vi "DoE_Control_v6.vi"() -> ()   [LabVIEW 2015]
uses:
  --Sensor and Instrument Drivers--/LabView VI Drivers for Heise DXD Digital Pressure Transducer/Type Defs/DXD Address.ctl
  --Controls and TypeDefs--/DoE_Control_Cluster.ctl
panel:
  out "Data Cluster 2":T1={"Current DoE"=[], "SSI 1 Flow Rate"=0.0, "SSI 2 Flow Rate"=0.0, "FLOM 1 Flow Rate"=0.0, "FLOM 2 Flow Rate"=0.0, "Pumps Running?"=FALSE, "Boolean 2"=FALSE, "Boolean 3"=FALSE, "Boolean 4"=FALSE, "At Equilibrium?"=FALSE, "Script Running?"=FALSE, "Current Script Iteration"=0.0, "Total Script Iterations"=0.0, "FLOM Pumps VISA"="COM2", "SSI 1 Pump VISA"="COM76", "SSI 2 Pump VISA"="COM74", "Huber Unistat VISA"="COM1", "SSI 3 Pump VISA"="COM76", "SSI 4 Pump VISA"="COM76", "SSI 4 Flow Rate"=0.0, "SSI 3 Flow Rate"=0.0, "Flow Meter 1"="COM76", "Flow Meter 2"="COM76", "Flow Meter 3"="COM76", "Flow Meter 4"="COM76", "Flow Meter 1 Rate "=0.0, "Flow Meter 2 Rate"=0.0, "Flow Meter 3 Rate"=0.0, "Flow Meter 4 Rate"=0.0, "SSI 1 Flow Setpoint"=0.0, "SSI 2 Flow Setpoint"=0.0, "SSI 3 Flow Setpoint"=0.0, "SSI 4 Flow Setpoint"=0.0, "Temperature Setpoint"=0.0} {"Current DoE" format="%0.3f"}
  in  "Sensor Readouts":T2(tab)
  out "Thermocouple T-Plots":cluster{dbl, dbl, dbl}(graph)
  in  "Flow meter 1 COM":u16=15
  in  "Flow meter 2 COM":u16=16
  in  "Flow meter 4 COM":u16=19
  in  "Flow meter 5 COM":u16=18
  out "Flow Rate":T3(graph)
  in  "Flow meter 3 COM":u16=17
  out "Temp":T4(graph)
  out "Pressure":T5(graph)
  in  "Pressure COM":refnum<visa-resource-name>="COM6"
  in  "Unit":T6(ring)
  in  "Write to File?":bool
  in  "?":T7(tab)
  in  "Collect Spectra":bool
  out "Raman Spectrum":cluster{i32[], i32[]}[](graph)
  in  "Reset?":bool
  in  "Cancel Script":bool
  in  "Data Cluster":T1={"Current DoE"=[], "SSI 1 Flow Rate"=0.0, "SSI 2 Flow Rate"=0.0, "FLOM 1 Flow Rate"=0.0, "FLOM 2 Flow Rate"=0.0, "Pumps Running?"=FALSE, "Boolean 2"=FALSE, "Boolean 3"=FALSE, "Boolean 4"=FALSE, "At Equilibrium?"=FALSE, "Script Running?"=FALSE, "Current Script Iteration"=0.0, "Total Script Iterations"=0.0, "FLOM Pumps VISA"="COM2", "SSI 1 Pump VISA"="COM76", "SSI 2 Pump VISA"="COM74", "Huber Unistat VISA"="COM1", "SSI 3 Pump VISA"="COM76", "SSI 4 Pump VISA"="COM76", "SSI 4 Flow Rate"=0.0, "SSI 3 Flow Rate"=0.0, "Flow Meter 1"="COM76", "Flow Meter 2"="COM76", "Flow Meter 3"="COM76", "Flow Meter 4"="COM76", "Flow Meter 1 Rate "=0.0, "Flow Meter 2 Rate"=0.0, "Flow Meter 3 Rate"=0.0, "Flow Meter 4 Rate"=0.0, "SSI 1 Flow Setpoint"=0.0, "SSI 2 Flow Setpoint"=0.0, "SSI 3 Flow Setpoint"=0.0, "SSI 4 Flow Setpoint"=0.0, "Temperature Setpoint"=0.0} {"Current DoE" format="%0.3f"}
  in  "?":T8(tab)
  in  "Huber Unistat VISA":refnum<visa-resource-name>="COM1"
  in  "SSI 4 Pump VISA":refnum<visa-resource-name>="COM10"
  in  "SSI 2 Pump VISA 2":refnum<visa-resource-name>="COM8"
  in  "SSI 1 Pump VISA":refnum<visa-resource-name>="COM7"
  in  "FLOM Pumps VISA":refnum<visa-resource-name>="LPT1"
  in  "SSI 3 Pump VISA":refnum<visa-resource-name>="COM9"
  in  "Set COMs":bool
  out "Data_noRaman path":path caption="selected path"
  out "Data_Reactant 1 path":path caption="selected path"
  out "Data_Product path":path caption="selected path"
  out "Data_Reactant 3 path":path caption="selected path"
  out "Data_Reactant 2 path":path caption="selected path"
  out "Raman Data Path":T9
  in  "Create DoE":bool
  out "file write cancelled":bool caption="cancelled"
  out "written file already exists (and overwritten)":bool caption="exists"
  in  "Input DoE Values":string[][](table)
  in  "Load DoE":bool
  out "Current DoE":dbl[][](array[numeric]) format="%0.3f"
  out "DoE Filename":path
  in  "Get Current DoE":bool
  in  "Stop-Start SSI 4":bool
  in  "Stop-Start SSI 3":bool
  in  "Edit or Run/Stop SSI 4":string(combo)="Run/Stop"
  in  "Edit or Run/Stop SSI 3":string(combo)="Run/Stop"
  in  "Pump 4 (Green)?":bool
  in  "Pump 3 (Yellow)?":bool
  in  "SSI  4 (Green)":dbl
  in  "SSI  3 (Yellow)":dbl
  in  "SSI  1 (Red)":dbl
  in  "Manual Pump Control?":bool
  in  "SSI  2 (Blue)":dbl
  in  "Pump 1 (Red)?":bool
  in  "Pump 2 (Blue)?":bool
  in  "Edit or Run/Stop SSI 2":string(combo)="Run/Stop"
  in  "Edit or Run/Stop SSI 1":string(combo)="Run/Stop"
  in  "Stop-Start SSI 1":bool
  in  "Stop-Start SSI 2":bool
  in  "FLOM 1":dbl min=0.0 max=9900.0 step=1.0
  in  "FLOM 2":dbl min=0.0 max=9900.0 step=1.0
  in  "FLOM 1?":bool
  in  "FLOM 2?":bool
  in  "Stop   Start FLOM 1":bool
  in  "Stop   Start FLOM 2":bool
  in  "Edit Values, or Run Flow? FLOM 2":string(combo)="Run/Stop"
  in  "Edit Values, or Run Flow? FLOM 1":string(combo)="Run/Stop"
  out "SSI  2  (Blue) Feedback":i32 format="%.2f"
  out "SSI  1  (Red) Feedback":i32 format="%.2f"
  out "SSI  3  (Yellow) Feedback":i32 format="%.2f"
  out "SSI  4  (Green) Feedback":i32 format="%.2f"
  in  "Set Temp / Lower Limit / Upper Limit":dbl
  in  "Manual Temp Control?":bool
  out "Last Command Written":string="Upper limit is"
  out "Temperature Output":string="Upper limit is"
  out "Last Message from Pump":string="Heating pump message, 2:38:53 PM:\nTemperature is set to 0.000000K"
  out "Error Out":T10
  in  "Commands":string(combo)="Setup"
  in  "Run Current DoE":bool
  out "Last Message from Pump":string="Heating pump message, 2:38:53 PM:\nTemperature is set to 0.000000K"
  out "Current Experiment":dbl[](array[numeric])
  in  "Debugging / Send Command":string
  in  "Debug":bool
  out "Program State":string
  in  "?":bool
  # "Most recent update: 2/23/2016 - JMW"
  # "Features To-Implement:\n\n- Yield Plotting and Analytics\n- Feedback Control based on Yield\n- Error Generation System\n     - for system and user safety"
  # "Notes:\n- set upper and lower temperature limits using \"Manual Temp Control\" \n     - DoE can't access T values outside of these limits\n- repeatedly turning the temperature control on and off can lead to compressor wear - avoid!\n- Added T and P readouts and saving\n- Always use Stop Program rather than the LabView stop button, else the Sensirion DLL\n   calls will error out and LabView must be restarted"
  # "Not corrrect com, set later"
  # "SSI 1"
  # "SSI 2"
  # "SSI 3"
  # "SSI 4"
  # "Temp"
  # "Time"
  # "FLOM 1"
  # "FLOM 2"
  # "SSI 1"
  # "SSI 2"
  # "SSI 3"
  # "SSI 4"
  # "FLOM 1"
  # "FLOM 2"
  # "Temp"
  # "Time"
  # "All flow rates in increments of 10uL/min"
  # "Note: don't repeatedly turn off and on temperature control as this can wear out the compressor too rapidly according to Unistat\nManual"
  # "Time"
  # "Temp"
  # "SSI 1"
  # "SSI 2"
  # "SSI 3"
  # "SSI 4"
  # "FLOM 1"
  # "FLOM 2"
  # "uL/min , degrees C, seconds"
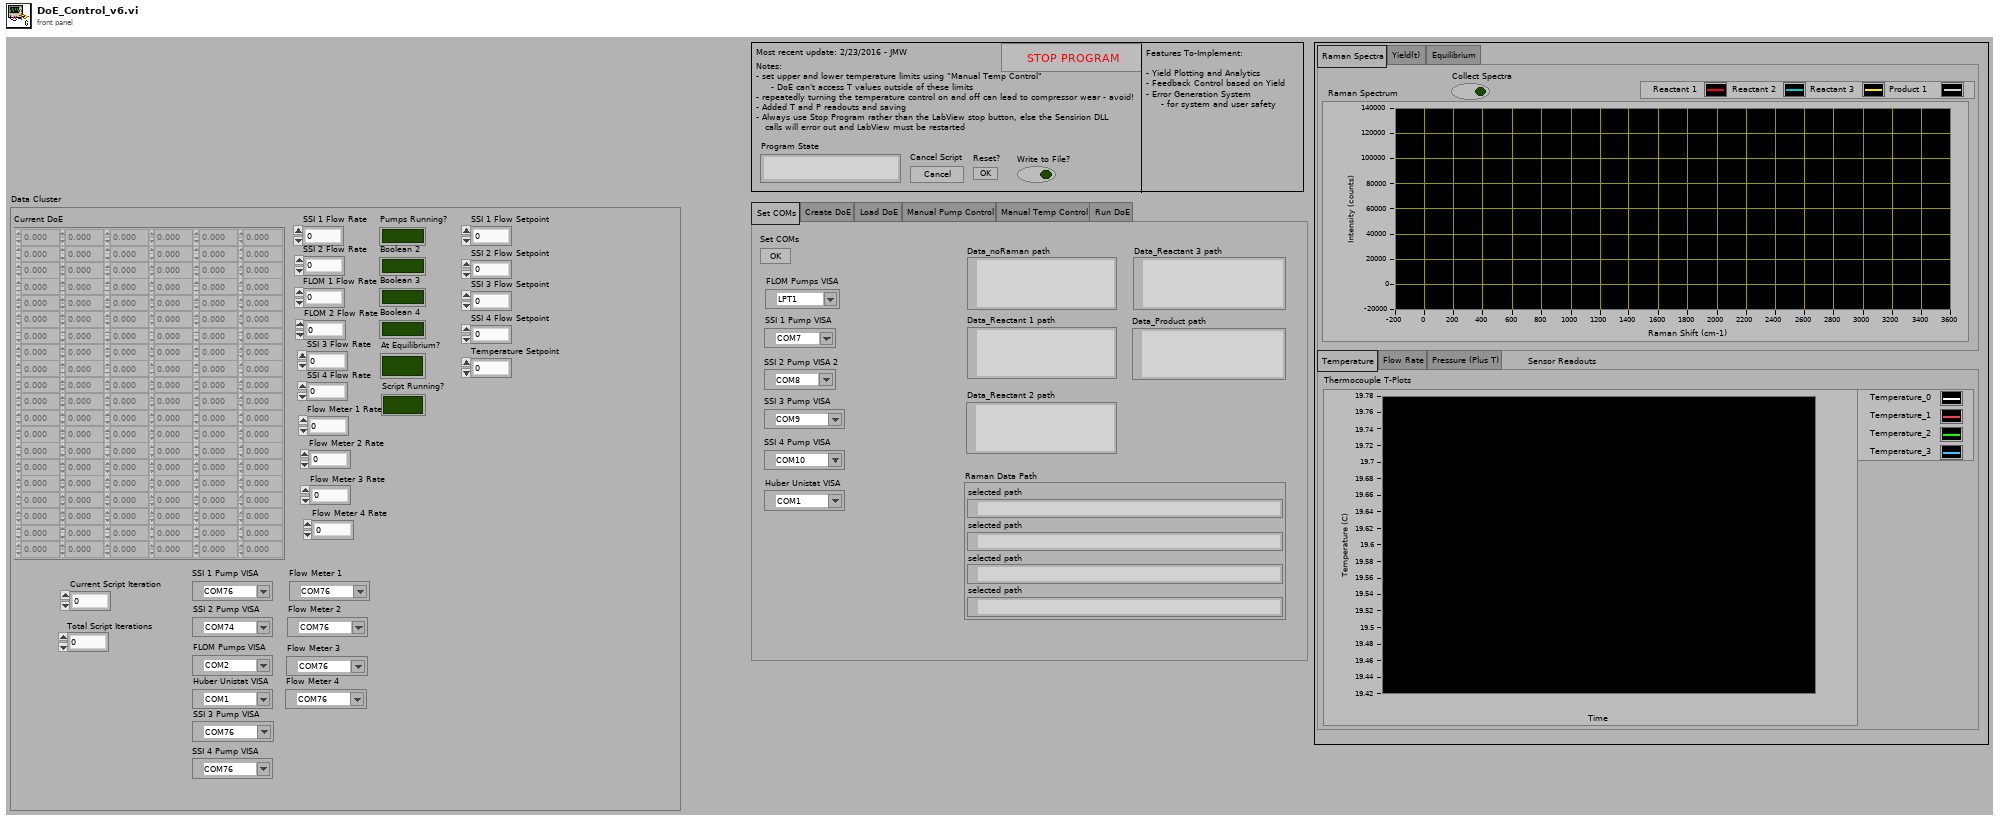
[diagram p1: front panel]
types:
  T1 = typedef "DoE_Control_Cluster.ctl" = cluster{"Current DoE":dbl[][], "SSI 1 Flow Rate":dbl, "SSI 2 Flow Rate":dbl, "FLOM 1 Flow Rate":dbl, "FLOM 2 Flow Rate":dbl, "Pumps Running?":bool, "Boolean 2":bool, "Boolean 3":bool, "Boolean 4":bool, "At Equilibrium?":bool, "Script Running?":bool, "Current Script Iteration":dbl, "Total Script Iterations":dbl, "FLOM Pumps VISA":refnum<visa-resource-name>, "SSI 1 Pump VISA":refnum<visa-resource-name>, "SSI 2 Pump VISA":refnum<visa-resource-name>, "Huber Unistat VISA":refnum<visa-resource-name>, "SSI 3 Pump VISA":refnum<visa-resource-name>, "SSI 4 Pump VISA":refnum<visa-resource-name>, "SSI 4 Flow Rate":dbl, "SSI 3 Flow Rate":dbl, "Flow Meter 1":refnum<visa-resource-name>, "Flow Meter 2":refnum<visa-resource-name>, "Flow Meter 3":refnum<visa-resource-name>, "Flow Meter 4":refnum<visa-resource-name>, "Flow Meter 1 Rate ":dbl, "Flow Meter 2 Rate":dbl, "Flow Meter 3 Rate":dbl, "Flow Meter 4 Rate":dbl, "SSI 1 Flow Setpoint":dbl, "SSI 2 Flow Setpoint":dbl, "SSI 3 Flow Setpoint":dbl, "SSI 4 Flow Setpoint":dbl, "Temperature Setpoint":dbl}
  T2 = enum32{"Temperature", "Flow Rate", "Pressure (Plus T)"}
  T3 = cluster{"MeasureResult Scaled":dbl, "MeasureResult Scaled":dbl, "MeasureResult Scaled":dbl, "MeasureResult Scaled":dbl, "MeasureResult Scaled":dbl}
  T4 = cluster{"Current Temperature":dbl, "Current Temperature":dbl, "Current Temperature":dbl, "Current Temperature":dbl}
  T5 = cluster{"Current Pressure":dbl, "Current Pressure":dbl, "Current Pressure":dbl, "Current Pressure":dbl}
  T6 = enum16{"PSI", "Bar", "cm H2O", "ft H2O", "hectoPascal", "in Hg", "in H2O", "kiloPascal", "milliBar", "mmHg", "MegaPascal", "Numeric Pressure"}
  T7 = enum32{"Raman Spectra", "Yield(t)", "Equilibrium"}
  T8 = enum32{"Set COMs", "Create DoE", "Load DoE", "Manual Pump Control", "Manual Temp Control", "Run DoE"}
  T9 = cluster{"selected path":path, "selected path":path, "selected path":path, "selected path":path}
  T10 = cluster{"status":bool, "code":i32, "Error Report":string}
  T11 = cluster{"Array":dbl[], "Array 2":dbl[], "Array 3":dbl[], "Array 4":dbl[], "Array 5":dbl[]}
  T12 = cluster{"MeasureResult Scaled":dbl, "MeasureResult Scaled":dbl, "MeasureResult Scaled":dbl, "MeasureResult Scaled":dbl, "MeasureResult Scaled":dbl}[]
  T13 = cluster{"appended path":path, "appended path":path, "appended path":path, "appended path":path, "appended path":path}
  T14 = cluster{"Current Pressure":dbl, "Current Pressure":dbl, "Current Pressure":dbl, "Current Pressure":dbl}[]
  T15 = cluster{"Current Temperature":dbl, "Current Temperature":dbl, "Current Temperature":dbl, "Current Temperature":dbl}[]
  T16 = typedef "DXD Address.ctl" = i32
  T17 = cluster{"Data_noRaman path":path, "Data_Reactant 1 path":path, "Data_Reactant 2 path":path, "Data_Reactant 3 path":path, "Data_Product path":path}
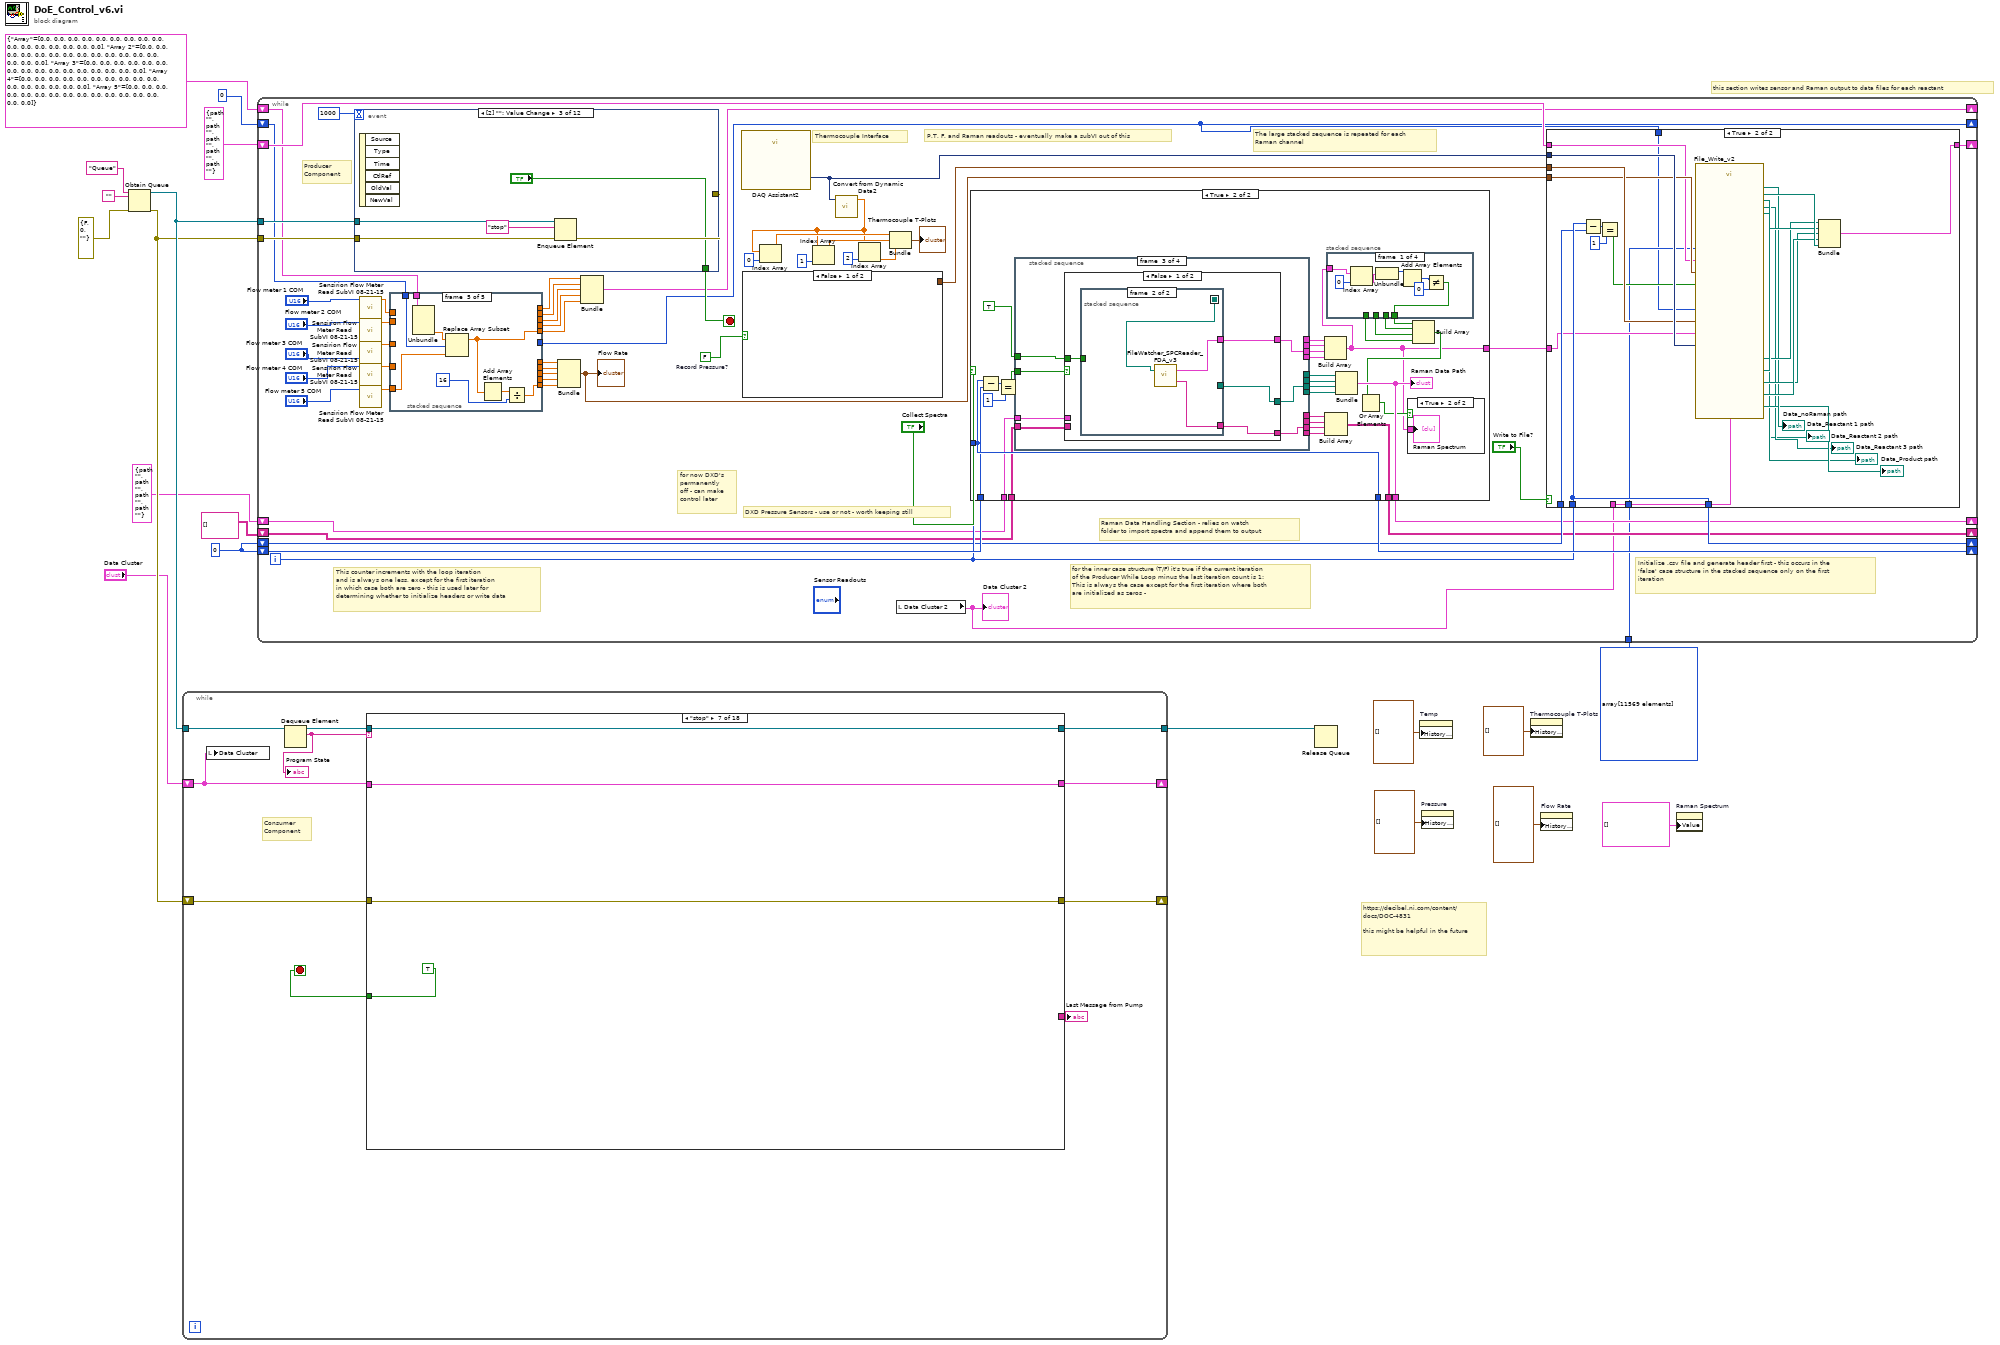
[diagram p0: block diagram]
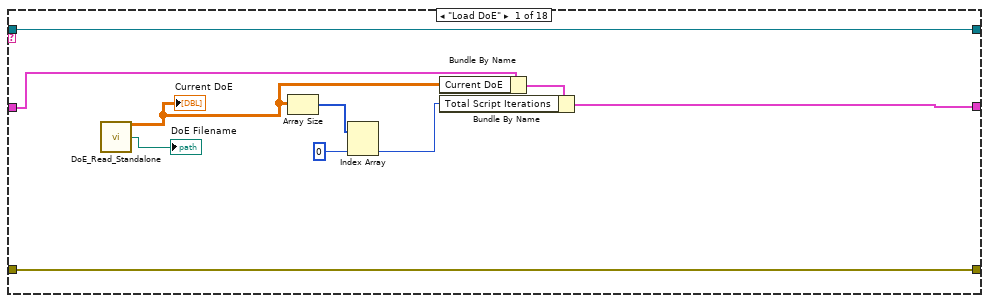
[diagram p2: hidden frame]
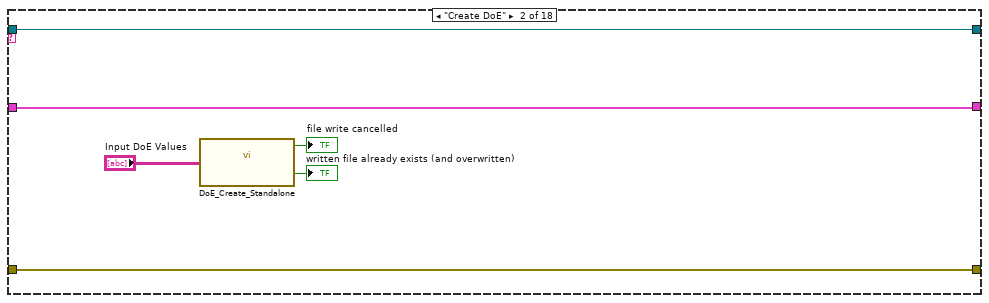
[diagram p3: hidden frame]
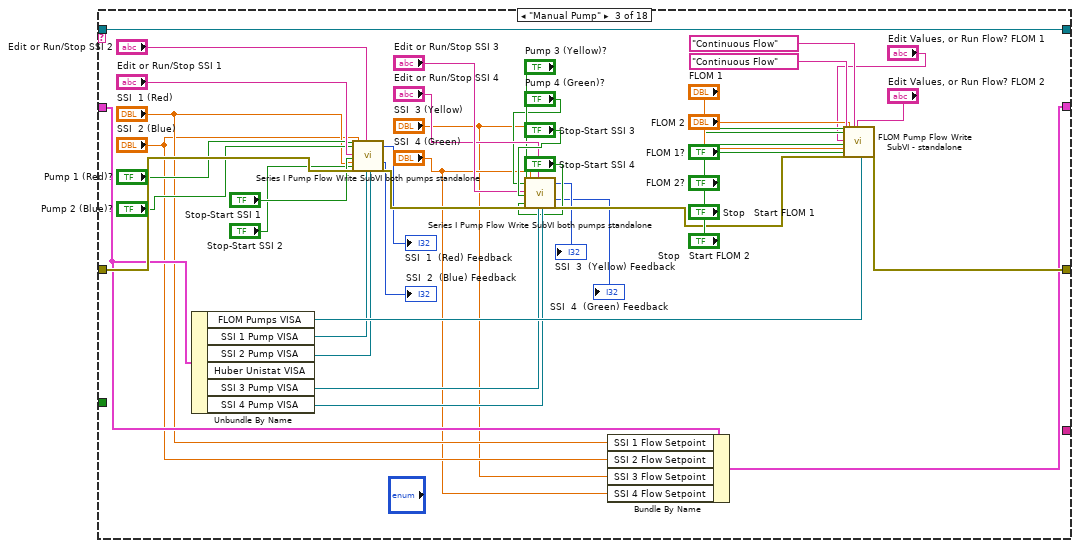
[diagram p4: hidden frame]
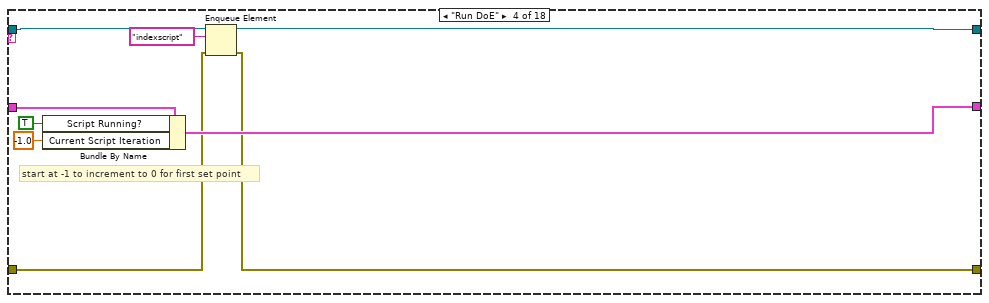
[diagram p5: hidden frame]
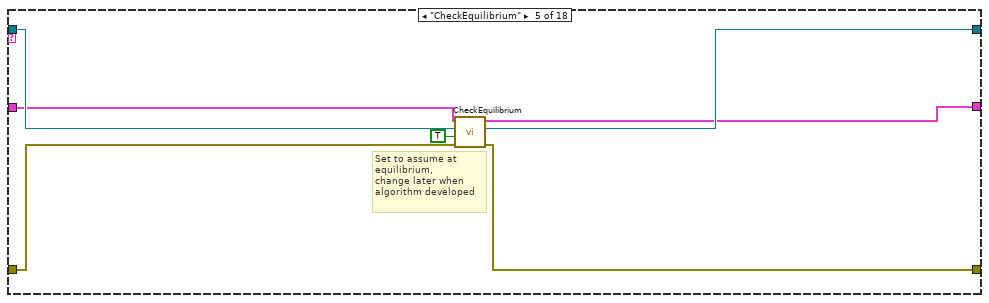
[diagram p6: hidden frame]
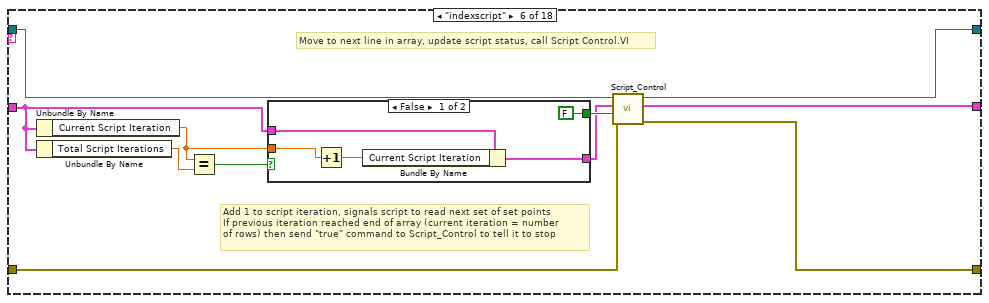
[diagram p7: hidden frame]
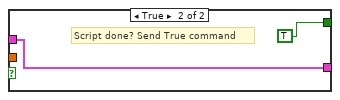
[diagram p8: hidden frame]
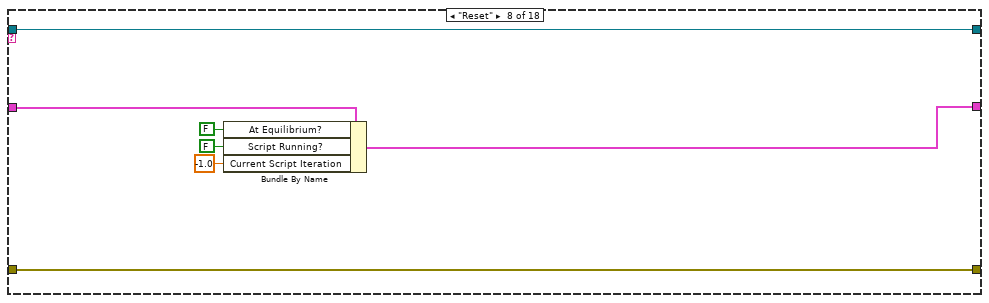
[diagram p9: hidden frame]
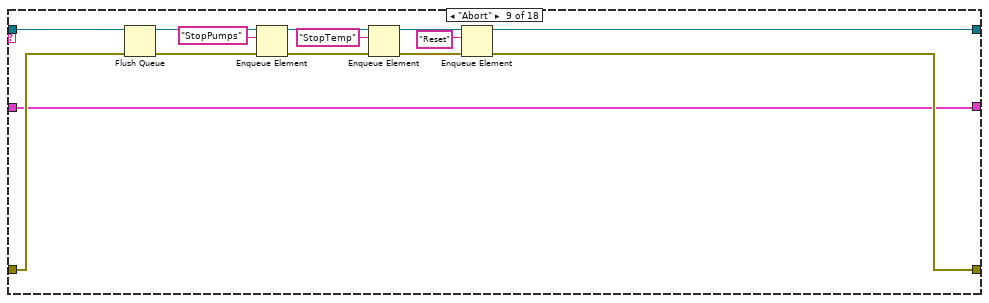
[diagram p10: hidden frame]
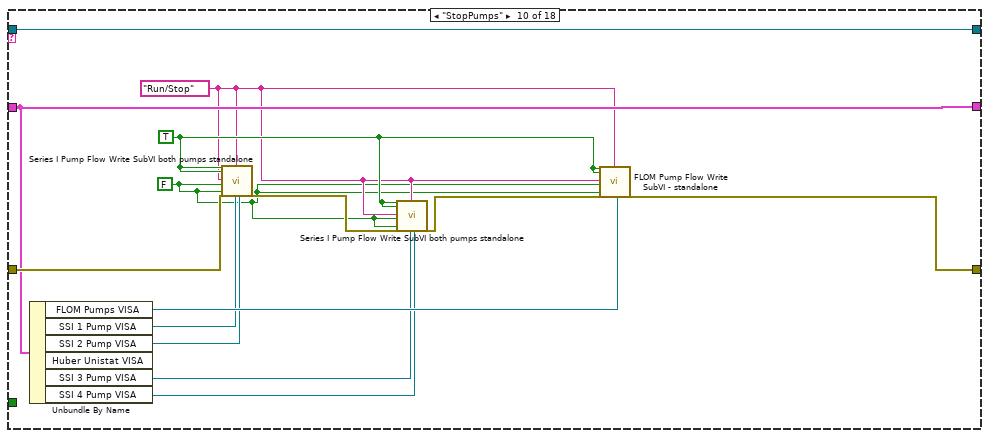
[diagram p11: hidden frame]
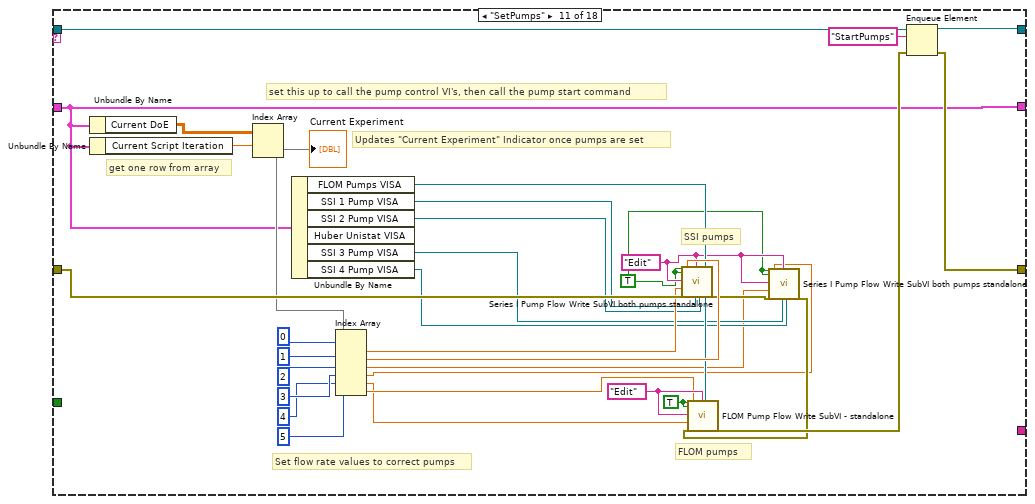
[diagram p12: hidden frame]
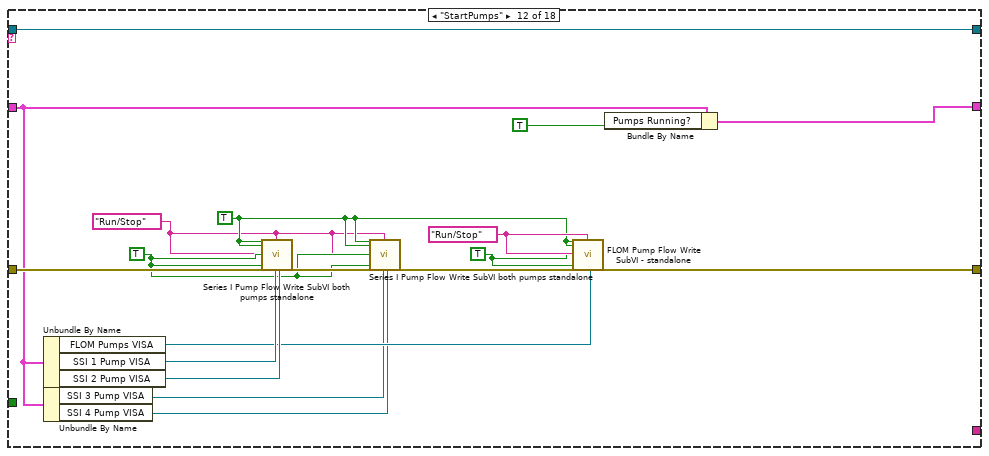
[diagram p13: hidden frame]
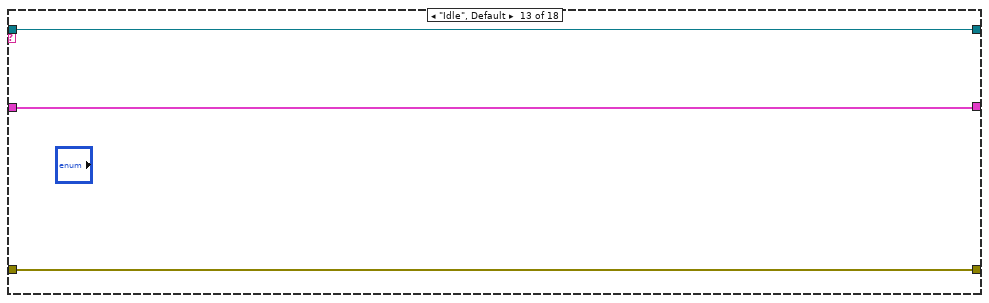
[diagram p14: hidden frame]
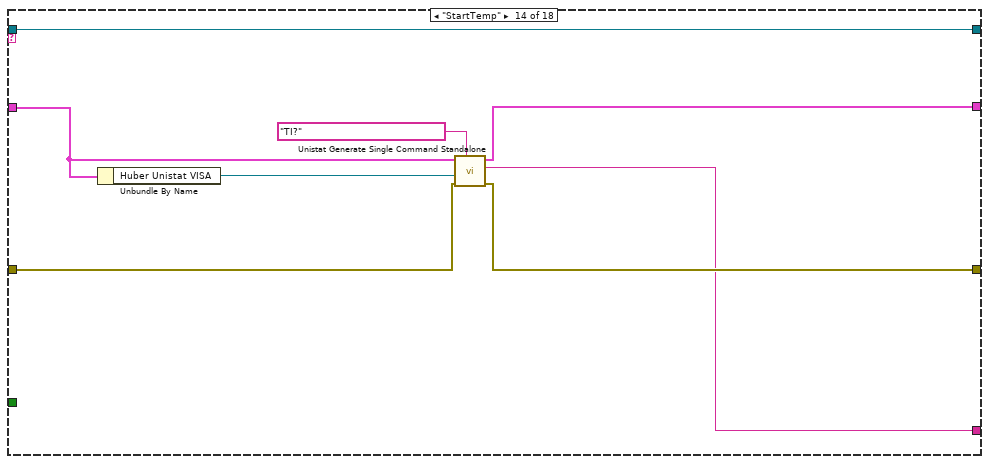
[diagram p15: hidden frame]
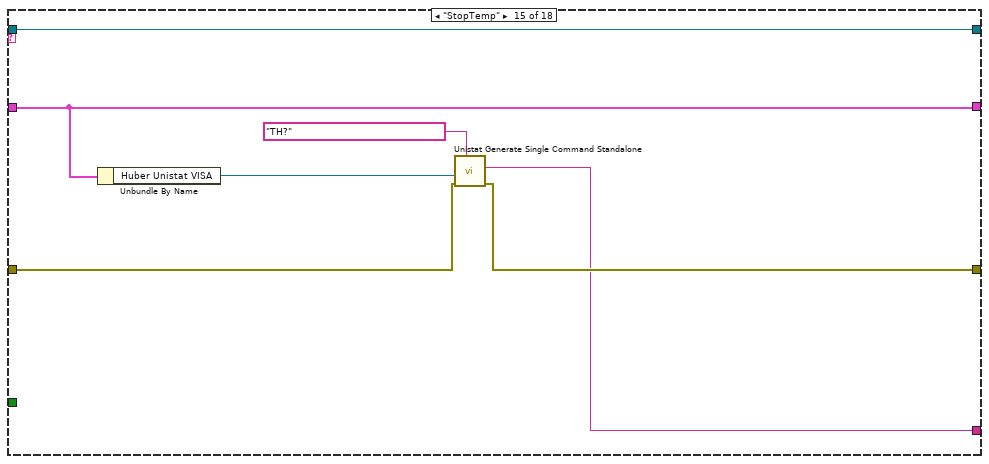
[diagram p16: hidden frame]
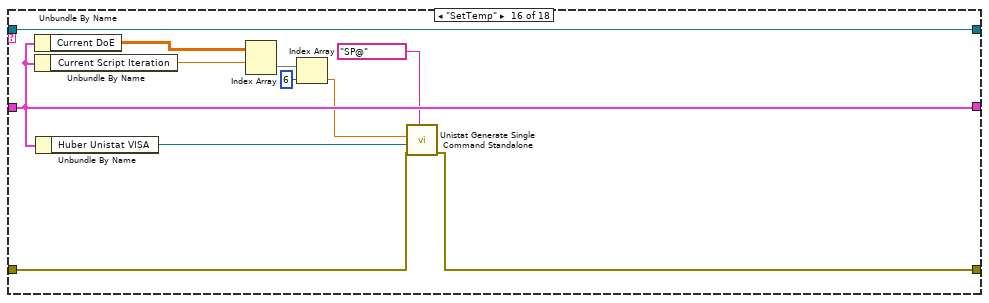
[diagram p17: hidden frame]
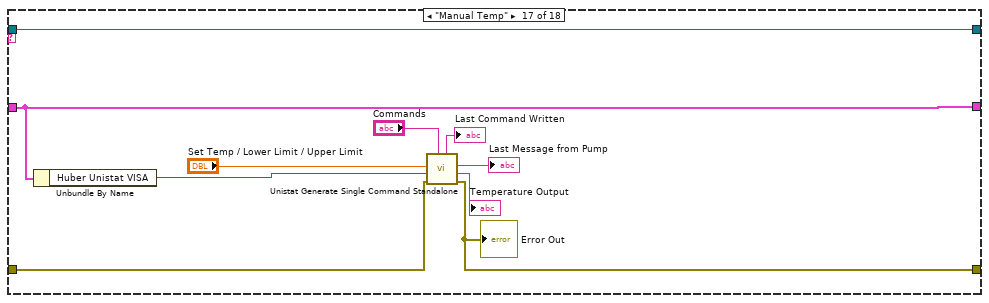
[diagram p18: hidden frame]
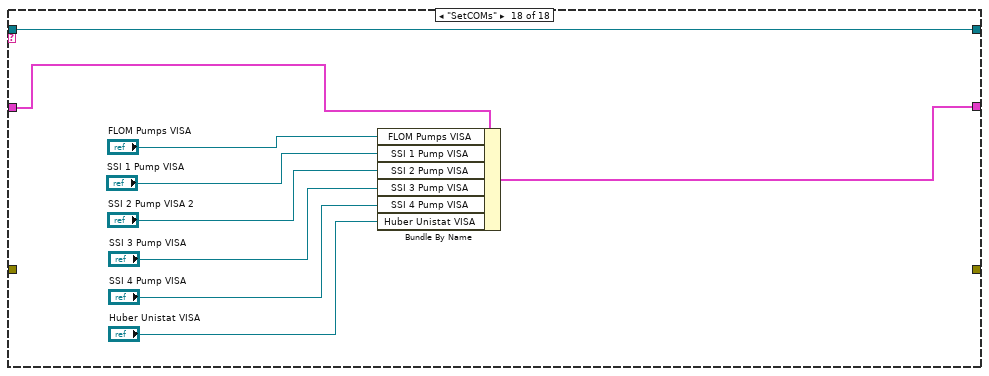
[diagram p19: hidden frame]
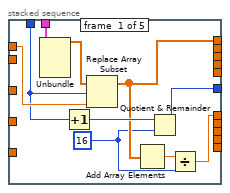
[diagram p20: hidden frame]
diagram:
  w10 = 0
  # "this section writes sensor and Raman output to data files for each reactant"
  # "https://decibel.ni.com/content/docs/DOC-4831\n\nthis might be helpful in the future"
  n1 = Obtain Queue(name (unnamed)="Queue", element data type="", error in (no error)=errorcluster {"status"=FALSE, "code"=0, "source"=""}) -> (queue out=w17:refnum<queue>, error out=w15:errorcluster)  [unwired: 2 in, 1 out]
  n2 = while {
    shift-right: [w26] -> _
    shift-left: w15 -> [w27]
    shift-right: [w23] -> _
    shift-left: "Data Cluster" -> [w20]
    tunnel: w17 -> [w28]
    tunnel: [w24] -> w14
    stop <- w21 stop-if-true
    # "Consumer \nComponent"
    n3 = local write "Data Cluster"(w20) -> ()
    n4 = Dequeue Element(queue=w28) -> (queue out=w25:refnum<queue>, element=w29:string)  [unwired: 2 in, 2 out]
    "Program State" <- w29
    n5 = case shown="\"stop\"" w29 {
      tunnel: w27 -> [w37 w40 w87 w92 w103 w112 w123 w132 w145 w159 w193 w210 w212 w221 w228 w239 w249 _]
      tunnel: [w37 w40 w69 w91 w102 w111 w123 w132 w135 w158 w176 w209 w212 w220 w227 w238 w248 _] -> w26
      tunnel: w20 -> [w38 w41 w51 w96 w98 w110 w124 w130 w133 w154 w173 w201 w214 w216 w226 w236 w246 w257]
      tunnel: [w32 w41 w46 w93 w97 w105 w124 w128 w133 w154 w173 w203 w214 w215 w226 w236 w246 w259] -> w23
      tunnel: [w36 w42 w70 w88 w101 w113 w125 w131 w134 w160 w177 w211 w213 w222 w229 w240 w247 w258] -> w24
      tunnel: w25 -> [w36 w42 w70 w90 w100 w114 w125 w131 w146 w160 w180 w211 w213 w222 w229 w240 w247 w258]
      tunnel: [_ _ _ _ _ _ _ _ _ _ _ _ _ w217 w223 _ _ _] -> w22
      tunnel: [_ _ _ _ _ _ TRUE _ _ _ _ _ _ _ _ _ _ _] -> w21
      frame "Load DoE" {
        n6 = call "DoE_Read_Standalone.vi"() -> ("all rows"=w35:dbl[][], "new file path (Not A Path if cancelled)"=→"DoE Filename":path)  [unwired: 14 in]
        "Current DoE" <- w35
        n7 = Array Size(array=w35) -> (size(s)=w33:i32[])
        n8 = Index Array(array=w33, index #2=0 ("index")) -> (element #2=w31:i32)  [unwired: 1 in, 1 out]
        n9 = Bundle By Name(cluster=w38, "Current DoE"=w35) -> (w34:T1)
        n10 = Bundle By Name(cluster=w34, "Total Script Iterations"=w31) -> (w32:T1)
      }
      frame "Create DoE" {
        n11 = call "DoE_Create_Standalone.vi"("Input DoE Values"="Input DoE Values") -> ("written file already exists (and overwritten)"=→"written file already exists (and overwritten)":bool, "file write cancelled"=→"file write cancelled":bool)  [unwired: 9 in]
      }
      frame "Manual Pump" {
        n12 = Unbundle By Name(w51) -> ("FLOM Pumps VISA"=w68:refnum<visa-resource-name>, "SSI 1 Pump VISA"=w67:refnum<visa-resource-name>, "SSI 2 Pump VISA"=w66:refnum<visa-resource-name>, "SSI 3 Pump VISA"=w63:refnum<visa-resource-name>, "SSI 4 Pump VISA"=w62:refnum<visa-resource-name>)  [unwired: 1 out]
        n13 = call "Series I Pump Flow Write SubVI both pumps standalone.vi"("Write to Pump 1?"="Pump 1 (Red)?", "Write to Pump 2?"="Pump 2 (Blue)?", "Edit or Run/Stop Series IA Pump"="Edit or Run/Stop SSI 1", "Stop-Start"="Stop-Start SSI 1", "Pump IA Flow Rate (10uL/min)"="SSI  1 (Red)", "Stop-Start 2"="Stop-Start SSI 2", "error in (no error)"=w87, "Pump 1B Flow Rate (10uL/min)"="SSI  2 (Blue)", "Edit or Run/Stop Series IB Pump"="Edit or Run/Stop SSI 2", "Series IA Pump VISA"=w67, "Series IB Pump VISA"=w66) -> ("Pump 1A flow rate Out"=→"SSI  1  (Red) Feedback":i32, "Pump 1B flow rate Out"=→"SSI  2  (Blue) Feedback":i32, "Error Out"=w65:T10)  [unwired: 13 in, 1 out]
        n14 = call "Series I Pump Flow Write SubVI both pumps standalone.vi"("Write to Pump 1?"="Pump 3 (Yellow)?", "Write to Pump 2?"="Pump 4 (Green)?", "Edit or Run/Stop Series IA Pump"="Edit or Run/Stop SSI 3", "Stop-Start"="Stop-Start SSI 3", "Pump IA Flow Rate (10uL/min)"="SSI  3 (Yellow)", "Stop-Start 2"="Stop-Start SSI 4", "error in (no error)"=w65, "Pump 1B Flow Rate (10uL/min)"="SSI  4 (Green)", "Edit or Run/Stop Series IB Pump"="Edit or Run/Stop SSI 4", "Series IA Pump VISA"=w63, "Series IB Pump VISA"=w62) -> ("Pump 1A flow rate Out"=→"SSI  3  (Yellow) Feedback":i32, "Pump 1B flow rate Out"=→"SSI  4  (Green) Feedback":i32, "Error Out"=w64:T10)  [unwired: 13 in, 1 out]
        n15 = Bundle By Name(cluster=w51, "SSI 1 Flow Setpoint"="SSI  1 (Red)", "SSI 2 Flow Setpoint"="SSI  2 (Blue)", "SSI 3 Flow Setpoint"="SSI  3 (Yellow)", "SSI 4 Flow Setpoint"="SSI  4 (Green)") -> (w46:T1)
        n16 = call "FLOM Pump Flow Write SubVI - standalone.vi"("Write to Pump 1?"="FLOM 1?", "Write to Pump 2?"="FLOM 2?", "Mode"="Continuous Flow", "Edit Values, or Run Flow?\n(Only for Continuous Flow)"="Edit Values, or Run Flow? FLOM 1", "Stop   Start"="Stop   Start FLOM 1", "Pump 1 Flow Rate (uL/min)"="FLOM 1", "Stop   Start 2"="Stop   Start FLOM 2", "error in (no error) 2"=w64, "Pump 2 Flow Rate (uL/min)"="FLOM 2", "Mode 2"="Continuous Flow", "Edit Values, or Run Flow?\n(Only for Continuous Flow) 2"="Edit Values, or Run Flow? FLOM 2", "VISA resource"=w68) -> ("Error Out"=w69:T10)  [unwired: 14 in, 1 out]
      }
      frame "Run DoE" {
        # "start at -1 to increment to 0 for first set point"
        n17 = Bundle By Name(cluster=w96, "Script Running?"=TRUE, "Current Script Iteration"=-1.0) -> (w93:T1)
        n18 = Enqueue Element(queue=w90, element="indexscript", error in (no error)=w92) -> (queue out=w88:refnum<queue>, error out=w91:errorcluster)  [unwired: 1 in, 1 out]
      }
      frame "CheckEquilibrium" {
        # "Set to assume at\nequilibrium,\nchange later when\nalgorithm developed"
        n19 = call "CheckEquilibrium.vi"("error in (no error)"=w103, "Eventually replace this with output from an algorithm to check equilibrium"=TRUE, "queue in"=w100, "Data Cluster"=w98) -> ("error out"=w102:errorcluster, "queue out"=w101:refnum<queue>, "Data Cluster 2"=w97:T1)  [unwired: 5 in]
      }
      frame "indexscript" {
        # "Add 1 to script iteration, signals script to read next set of set points\nIf previous iteration reached end of array (current iteration = number\nof rows) then send \"true\" command to Script_Control to tell it to stop"
        # "Move to next line in array, update script status, call Script Control.VI"
        n20 = Unbundle By Name(w110) -> ("Current Script Iteration"=w107:dbl)
        n21 = Unbundle By Name(w110) -> ("Total Script Iterations"=w108:dbl)
        n22 = Equal?(x=w107, y=w108) -> (x = y?=w104:bool)
        n23 = case shown="False" w104 {
          tunnel: w107 -> [w119 _]
          tunnel: w110 -> [w117 w121]
          tunnel: [w116 w121] -> w106
          tunnel: [FALSE TRUE] -> w109
          frame False {
            n24 = Increment(x=w119) -> (x+1=w118:dbl)
            n25 = Bundle By Name(cluster=w117, "Current Script Iteration"=w118) -> (w116:T1)
          }
          frame True {
            # "Script done? Send True command"
          }
        }
        n26 = call "Script_Control.vi"("error in (no error)"=w112, "Script done? Replace later"=w109, "Data Cluster"=w106, "queue in"=w114) -> ("error out"=w111:errorcluster, "Data Cluster 2"=w105:T1, "queue out"=w113:refnum<queue>)  [unwired: 5 in]
      }
      frame "stop" {
      }
      frame "Reset" {
        n27 = Bundle By Name(cluster=w130, "At Equilibrium?"=FALSE, "Script Running?"=FALSE, "Current Script Iteration"=-1.0) -> (w128:T1)
      }
      frame "Abort" {
        n28 = Flush Queue(queue=w146, error in (no error)=w145) -> (queue out=w144:refnum<queue>, error out=w143:errorcluster)  [unwired: 1 out]
        n29 = Enqueue Element(queue=w144, element="StopPumps", error in (no error)=w143) -> (queue out=w141:refnum<queue>, error out=w142:errorcluster)  [unwired: 1 in, 1 out]
        n30 = Enqueue Element(queue=w141, element="StopTemp", error in (no error)=w142) -> (queue out=w137:refnum<queue>, error out=w138:errorcluster)  [unwired: 1 in, 1 out]
        n31 = Enqueue Element(queue=w137, element="Reset", error in (no error)=w138) -> (queue out=w134:refnum<queue>, error out=w135:errorcluster)  [unwired: 1 in, 1 out]
      }
      frame "StopPumps" {
        w150 = "Run/Stop" ("Edit or Run/Stop Series IB Pump")
        w149 = FALSE ("Stop-Start")
        w151 = TRUE ("Write to Pump 1?")
        n32 = Unbundle By Name(w154) -> ("FLOM Pumps VISA"=w157:refnum<visa-resource-name>, "SSI 1 Pump VISA"=w156:refnum<visa-resource-name>, "SSI 2 Pump VISA"=w155:refnum<visa-resource-name>, "SSI 3 Pump VISA"=w148:refnum<visa-resource-name>, "SSI 4 Pump VISA"=w147:refnum<visa-resource-name>)  [unwired: 1 out]
        n33 = call "Series I Pump Flow Write SubVI both pumps standalone.vi"("Write to Pump 1?"=w151, "Write to Pump 2?"=w151, "Edit or Run/Stop Series IA Pump"=w150, "Stop-Start"=w149, "Stop-Start 2"=w149, "error in (no error)"=w159, "Edit or Run/Stop Series IB Pump"=w150, "Series IA Pump VISA"=w156, "Series IB Pump VISA"=w155) -> ("Error Out"=w153:T10)  [unwired: 15 in, 3 out]
        n34 = call "Series I Pump Flow Write SubVI both pumps standalone.vi"("Write to Pump 1?"=w151, "Write to Pump 2?"=w151, "Edit or Run/Stop Series IA Pump"=w150, "Stop-Start"=w149, "Stop-Start 2"=w149, "error in (no error)"=w153, "Edit or Run/Stop Series IB Pump"=w150, "Series IA Pump VISA"=w148, "Series IB Pump VISA"=w147) -> ("Error Out"=w152:T10)  [unwired: 15 in, 3 out]
        n35 = call "FLOM Pump Flow Write SubVI - standalone.vi"("Write to Pump 1?"=w151, "Write to Pump 2?"=w151, "Edit Values, or Run Flow?\n(Only for Continuous Flow)"=w150, "Stop   Start"=w149, "Stop   Start 2"=w149, "error in (no error) 2"=w152, "Edit Values, or Run Flow?\n(Only for Continuous Flow) 2"=w150, "VISA resource"=w157) -> ("Error Out"=w158:T10)  [unwired: 18 in, 1 out]
      }
      frame "SetPumps" {
        w174 = TRUE ("Write to Pump 1?")
        w175 = "Edit" ("Edit Values, or Run Flow?\n(Only for Continuous Flow)")
        w171 = TRUE ("Write to Pump 1?")
        w172 = "Edit" ("Edit or Run/Stop Series IB Pump")
        # "FLOM pumps"
        # "SSI pumps"
        # "Set flow rate values to correct pumps"
        # "get one row from array"
        # "set this up to call the pump control VI's, then call the pump start command"
        # "Updates \"Current Experiment\" Indicator once pumps are set"
        n36 = Unbundle By Name(w173) -> ("Current DoE"=w192:dbl[][])
        n37 = Unbundle By Name(w173) -> ("Current Script Iteration"=w191:dbl)
        n38 = Index Array(array=w192, index (row)=w191) -> (element=w190:dbl[])  [unwired: 1 in]
        "Current Experiment" <- w190
        n39 = Unbundle By Name(w173) -> ("FLOM Pumps VISA"=w181:refnum<visa-resource-name>, "SSI 1 Pump VISA"=w183:refnum<visa-resource-name>, "SSI 2 Pump VISA"=w182:refnum<visa-resource-name>, "SSI 3 Pump VISA"=w170:refnum<visa-resource-name>, "SSI 4 Pump VISA"=w169:refnum<visa-resource-name>)  [unwired: 1 out]
        n40 = Index Array(array=w190, index #1=0 ("index"), index #2=1 ("index"), index #3=2 ("index"), index #4=3 ("index"), index #5=4 ("index"), index #6=5 ("index")) -> (element #1=w185:dbl, element #2=w184:dbl, element #3=w164:dbl, element #4=w163:dbl, element #5=w161:dbl, element #6=w162:dbl)
        n41 = call "Series I Pump Flow Write SubVI both pumps standalone.vi"("Write to Pump 1?"=w171, "Write to Pump 2?"=w171, "Edit or Run/Stop Series IA Pump"=w172, "Pump IA Flow Rate (10uL/min)"=w185, "error in (no error)"=w193, "Pump 1B Flow Rate (10uL/min)"=w184, "Edit or Run/Stop Series IB Pump"=w172, "Series IA Pump VISA"=w183, "Series IB Pump VISA"=w182) -> ("Error Out"=w168:T10)  [unwired: 15 in, 3 out]
        n42 = call "Series I Pump Flow Write SubVI both pumps standalone.vi"("Write to Pump 1?"=w171, "Write to Pump 2?"=w171, "Edit or Run/Stop Series IA Pump"=w172, "Pump IA Flow Rate (10uL/min)"=w164, "error in (no error)"=w168, "Pump 1B Flow Rate (10uL/min)"=w163, "Edit or Run/Stop Series IB Pump"=w172, "Series IA Pump VISA"=w170, "Series IB Pump VISA"=w169) -> ("Error Out"=w167:T10)  [unwired: 15 in, 3 out]
        n43 = call "FLOM Pump Flow Write SubVI - standalone.vi"("Write to Pump 1?"=w174, "Write to Pump 2?"=w174, "Edit Values, or Run Flow?\n(Only for Continuous Flow)"=w175, "Pump 1 Flow Rate (uL/min)"=w161, "error in (no error) 2"=w167, "Pump 2 Flow Rate (uL/min)"=w162, "Edit Values, or Run Flow?\n(Only for Continuous Flow) 2"=w175, "VISA resource"=w181) -> ("Error Out"=w179:T10)  [unwired: 18 in, 1 out]
        n44 = Enqueue Element(queue=w180, element="StartPumps", error in (no error)=w179) -> (queue out=w177:refnum<queue>, error out=w176:errorcluster)  [unwired: 1 in, 1 out]
      }
      frame "StartPumps" {
        w197 = TRUE ("Stop-Start")
        w204 = TRUE ("Stop   Start")
        w205 = "Run/Stop" ("Edit Values, or Run Flow?\n(Only for Continuous Flow) 2")
        w196 = "Run/Stop" ("Edit or Run/Stop Series IB Pump")
        w198 = TRUE ("Write to Pump 1?")
        n45 = Unbundle By Name(w201) -> ("FLOM Pumps VISA"=w206:refnum<visa-resource-name>, "SSI 1 Pump VISA"=w208:refnum<visa-resource-name>, "SSI 2 Pump VISA"=w207:refnum<visa-resource-name>)
        n46 = Unbundle By Name(w201) -> ("SSI 3 Pump VISA"=w195:refnum<visa-resource-name>, "SSI 4 Pump VISA"=w194:refnum<visa-resource-name>)
        n47 = call "Series I Pump Flow Write SubVI both pumps standalone.vi"("Write to Pump 1?"=w198, "Write to Pump 2?"=w198, "Edit or Run/Stop Series IA Pump"=w196, "Stop-Start"=w197, "Stop-Start 2"=w197, "error in (no error)"=w210, "Edit or Run/Stop Series IB Pump"=w196, "Series IA Pump VISA"=w208, "Series IB Pump VISA"=w207) -> ("Error Out"=w200:T10)  [unwired: 15 in, 3 out]
        n48 = call "Series I Pump Flow Write SubVI both pumps standalone.vi"("Write to Pump 1?"=w198, "Write to Pump 2?"=w198, "Edit or Run/Stop Series IA Pump"=w196, "Stop-Start"=w197, "Stop-Start 2"=w197, "error in (no error)"=w200, "Edit or Run/Stop Series IB Pump"=w196, "Series IA Pump VISA"=w195, "Series IB Pump VISA"=w194) -> ("Error Out"=w199:T10)  [unwired: 15 in, 3 out]
        n49 = call "FLOM Pump Flow Write SubVI - standalone.vi"("Write to Pump 1?"=w198, "Write to Pump 2?"=w198, "Edit Values, or Run Flow?\n(Only for Continuous Flow)"=w205, "Stop   Start"=w204, "Stop   Start 2"=w204, "error in (no error) 2"=w199, "Edit Values, or Run Flow?\n(Only for Continuous Flow) 2"=w205, "VISA resource"=w206) -> ("Error Out"=w209:T10)  [unwired: 18 in, 1 out]
        n50 = Bundle By Name(cluster=w201, "Pumps Running?"=TRUE ("Boolean")) -> (w203:T1)
      }
      frame "Idle", Default {
      }
      frame "StartTemp" {
        n51 = Unbundle By Name(w216) -> ("Huber Unistat VISA"=w219:refnum<visa-resource-name>)
        n52 = call "Unistat Generate Single Command Standalone.vi"("Commands"="TI?", "error in (no error)"=w221, "VISA resource"=w219, "Data Cluster"=w216) -> ("Error Out"=w220:T10, "Last Message from Pump"=w217:string, "Data Cluster 2"=w215:T1)  [unwired: 3 in, 2 out]
      }
      frame "StopTemp" {
        n53 = Unbundle By Name(w226) -> ("Huber Unistat VISA"=w225:refnum<visa-resource-name>)
        n54 = call "Unistat Generate Single Command Standalone.vi"("Commands"="TH?", "error in (no error)"=w228, "VISA resource"=w225) -> ("Error Out"=w227:T10, "Last Message from Pump"=w223:string)  [unwired: 4 in, 3 out]
      }
      frame "SetTemp" {
        n55 = Unbundle By Name(w236) -> ("Current DoE"=w233:dbl[][])
        n56 = Unbundle By Name(w236) -> ("Current Script Iteration"=w234:dbl)
        n57 = Unbundle By Name(w236) -> ("Huber Unistat VISA"=w237:refnum<visa-resource-name>)
        n58 = Index Array(array=w233, index (row)=w234) -> (element=w232:dbl[])  [unwired: 1 in]
        n59 = Index Array(array=w232, index=6) -> (element=w231:dbl)
        n60 = call "Unistat Generate Single Command Standalone.vi"("Commands"="SP@", "error in (no error)"=w239, "VISA resource"=w237, "Temperature"=w231) -> ("Error Out"=w238:T10)  [unwired: 3 in, 4 out]
      }
      frame "Manual Temp" {
        n61 = Unbundle By Name(w246) -> ("Huber Unistat VISA"=w245:refnum<visa-resource-name>)
        n62 = call "Unistat Generate Single Command Standalone.vi"("Commands"="Commands", "error in (no error)"=w249, "VISA resource"=w245, "Temperature"="Set Temp / Lower Limit / Upper Limit") -> ("Error Out"=w248:T10, "Temperature Output"=→"Temperature Output":string, "Last Message from Pump"=→"Last Message from Pump":string, "Last Command Written"=→"Last Command Written":string)  [unwired: 3 in, 1 out]
        "Error Out" <- w248
      }
      frame "SetCOMs" {
        n63 = Bundle By Name(cluster=w257, "FLOM Pumps VISA"="FLOM Pumps VISA", "SSI 1 Pump VISA"="SSI 1 Pump VISA", "SSI 2 Pump VISA"="SSI 2 Pump VISA 2", "SSI 3 Pump VISA"="SSI 3 Pump VISA", "SSI 4 Pump VISA"="SSI 4 Pump VISA", "Huber Unistat VISA"="Huber Unistat VISA") -> (w259:T1)
      }
    }
    "Last Message from Pump" <- w22
  }
  n64 = while {
    tunnel: w17 -> [w315]
    tunnel: w15 -> [w314]
    shift-right: [w293] -> _
    shift-left: w10 -> [w294]
    shift-right: [w296] -> _
    shift-left: T13 {"appended path"=path "", "appended path"=path "", "appended path"=path "", "appended path"=path "", "appended path"=path ""} -> [w281]
    shift-right: [w292] -> _
    shift-left: w10 -> [w290]
    shift-right: [w286] -> _
    shift-left: string[][] [] -> [w285]
    shift-right: [w288] -> _
    shift-left: T9 {"selected path"=path "", "selected path"=path "", "selected path"=path "", "selected path"=path ""} -> [w287]
    tunnel: i32[] array[11569 elements] ("Array") -> [w284]
    shift-right: [w275] -> _
    shift-left: T11 {"Array"=[0.0, 0.0, 0.0, 0.0, 0.0, 0.0, 0.0, 0.0, 0.0, 0.0, 0.0, 0.0, 0.0, 0.0, 0.0, 0.0], "Array 2"=[0.0, 0.0, 0.0, 0.0, 0.0, 0.0, 0.0, 0.0, 0.0, 0.0, 0.0, 0.0, 0.0, 0.0, 0.0, 0.0], "Array 3"=[0.0, 0.0, 0.0, 0.0, 0.0, 0.0, 0.0, 0.0, 0.0, 0.0, 0.0, 0.0, 0.0, 0.0, 0.0, 0.0], "Array 4"=[0.0, 0.0, 0.0, 0.0, 0.0, 0.0, 0.0, 0.0, 0.0, 0.0, 0.0, 0.0, 0.0, 0.0, 0.0, 0.0], "Array 5"=[0.0, 0.0, 0.0, 0.0, 0.0, 0.0, 0.0, 0.0, 0.0, 0.0, 0.0, 0.0, 0.0, 0.0, 0.0, 0.0]} -> [w274]
    shift-right: [w261] -> _
    shift-left: 0 -> [w263]
    i -> [w291]
    stop <- w283 stop-if-true
    w310 = FALSE  # Record Pressure?
    # "Producer\nComponent"
    # "Initialize .csv file and generate header first - this occurs in the 'false' case structure in the stacked sequence only on the first iteration"
    # "The large stacked sequence is repeated for each\nRaman channel"
    # "for the inner case structure (T/F) it's true if the current iteration\nof the Producer While Loop minus the last iteration count is 1:\nThis is always the case except for the first iteration where both\nare initialized as zeros -"
    # "This counter increments with the loop iteration\nand is always one less, except for the first iteration\nin which case both are zero - this is used later for \ndetermining whether to initialize headers or write data"
    # "Raman Data Handling Section - relies on watch \nfolder to import spectra and append them to output"
    # "Thermocouple Interface"
    # "for now DXD's \npermanently\noff - can make\ncontrol later"
    # "DXD Pressure Sensors - use or not - worth keeping still"
    # "P,T, F, and Raman readouts - eventually make a subVI out of this"
    n65 = event shown="[2] \"\": Value Change" {
      selector: _ -> [_ _ _ _ _ _ _ _ _ _ _ _]
      dyn-events: _ -> [_ _ _ _ _ _ _ _ _ _ _ _]
      timeout: u32 1000 ("Time") -> [_ _ _ _ _ _ _ _ _ _ _ _]
      tunnel: w315 -> [w567 w570 w575 w581 w584 w589 w595 w598 w602 w607 w610 w614]
      tunnel: w314 -> [w568 w572 w577 w579 w585 w587 w594 w599 w601 w606 w611 w615]
      tunnel: [w565 w571 w576 w578 w582 w586 w590 w597 w600 w604 _ w613] -> _
      tunnel: [_ _ _ _ _ _ _ _ _ _ w609 _] -> _
      tunnel: [_ _ "?" _ _ _ _ _ _ _ _ _] -> w283
      event Timeout {
        n66 = event-data() -> ()  [unwired: 1 in, 2 out]
        n67 = Enqueue Element(queue=w567, element="Idle", error in (no error)=w568) -> (error out=w565:errorcluster)  [unwired: 1 in, 2 out]
      }
      event "Set COMs": Value Change {
        n68 = event-data() -> ()  [unwired: 1 in, 6 out]
        n69 = Enqueue Element(queue=w570, element="SetCOMs", error in (no error)=w572) -> (error out=w571:errorcluster)  [unwired: 1 in, 2 out]
      }
      event Value Change {
        n70 = event-data() -> ()  [unwired: 1 in, 6 out]
        n71 = Enqueue Element(queue=w575, element="stop", error in (no error)=w577) -> (error out=w576:errorcluster)  [unwired: 1 in, 2 out]
      }
      event "Run Current DoE": Value Change {
        n72 = event-data() -> ()  [unwired: 1 in, 5 out]
        n73 = Enqueue Element(queue=w581, element="Run DoE", error in (no error)=w579) -> (error out=w578:errorcluster)  [unwired: 1 in, 2 out]
      }
      event "Manual Pump Control?": Value Change {
        n74 = event-data() -> ()  [unwired: 1 in, 5 out]
        n75 = Enqueue Element(queue=w584, element="Manual Pump", error in (no error)=w585) -> (error out=w582:errorcluster)  [unwired: 1 in, 2 out]
      }
      event "Create DoE": Value Change {
        n76 = event-data() -> ()  [unwired: 1 in, 5 out]
        n77 = Enqueue Element(queue=w589, element="Create DoE", error in (no error)=w587) -> (error out=w586:errorcluster)  [unwired: 1 in, 2 out]
      }
      event "Cancel Script": Value Change {
        n78 = event-data() -> ()  [unwired: 1 in, 5 out]
        n79 = Flush Queue(queue=w595, error in (no error)=w594) -> (queue out=w593:refnum<queue>, error out=w592:errorcluster)  [unwired: 1 out]
        n80 = Enqueue Element(queue=w593, element="Abort", error in (no error)=w592) -> (error out=w590:errorcluster)  [unwired: 1 in, 2 out]
      }
      event "Manual Temp Control?": Value Change {
        n81 = event-data() -> ()  [unwired: 1 in, 5 out]
        n82 = Enqueue Element(queue=w598, element="Manual Temp", error in (no error)=w599) -> (error out=w597:errorcluster)  [unwired: 1 in, 2 out]
      }
      event "Load DoE": Value Change {
        n83 = event-data() -> ()  [unwired: 1 in, 5 out]
        n84 = Enqueue Element(queue=w602, element="Load DoE", error in (no error)=w601) -> (error out=w600:errorcluster)  [unwired: 1 in, 2 out]
      }
      event "Get Current DoE": Value Change {
        n85 = event-data() -> ()  [unwired: 1 in, 5 out]
        n86 = Enqueue Element(queue=w607, element="Get DoE", error in (no error)=w606) -> (error out=w604:errorcluster)  [unwired: 1 in, 2 out]
      }
      event "Debug": Value Change {
        n87 = event-data() -> ()  [unwired: 1 in, 5 out]
        n88 = Enqueue Element(queue=w610, element="Debugging / Send Command", error in (no error)=w611) -> (error out=w609:errorcluster)  [unwired: 1 in, 2 out]
      }
      event "Reset?": Value Change {
        n89 = event-data() -> ()  [unwired: 1 in, 5 out]
        n90 = Enqueue Element(queue=w614, element="Reset", error in (no error)=w615) -> (error out=w613:errorcluster)  [unwired: 1 in, 2 out]
      }
    }
    n91 = call "Sensirion Flow Meter Read SubVI 08-21-15.vi"("COMPort"="Flow meter 1 COM") -> ("MeasureResult Scaled"=w280:dbl)  [unwired: 10 in]
    n92 = call "Sensirion Flow Meter Read SubVI 08-21-15.vi"("COMPort"="Flow meter 2 COM") -> ("MeasureResult Scaled"=w267:dbl)  [unwired: 10 in]
    n93 = call "Sensirion Flow Meter Read SubVI 08-21-15.vi"("COMPort"="Flow meter 3 COM") -> ("MeasureResult Scaled"=w266:dbl)  [unwired: 10 in]
    n94 = call "Sensirion Flow Meter Read SubVI 08-21-15.vi"("COMPort"="Flow meter 4 COM") -> ("MeasureResult Scaled"=w265:dbl)  [unwired: 10 in]
    n95 = call "Sensirion Flow Meter Read SubVI 08-21-15.vi"("COMPort"="Flow meter 5 COM") -> ("MeasureResult Scaled"=w264:dbl)  [unwired: 10 in]
    n96 = stacked-sequence {
      tunnel: [w321 _ _ _ _] -> w278
      tunnel: w263 -> [w322 w333 w341 w349 w357]
      tunnel: [w324 _ _ _ _] -> w261
      tunnel: w280 -> [w323 _ _ _ _]
      tunnel: [w318 _ _ _ _] -> w279
      tunnel: w274 -> [w317 w328 w338 w346 w354]
      tunnel: [_ w330 _ _ _] -> w277
      tunnel: [_ w329 _ _ _] -> w276
      tunnel: [_ _ w337 _ _] -> w273
      tunnel: [_ _ w336 _ _] -> w272
      tunnel: [_ _ _ w345 _] -> w271
      tunnel: [_ _ _ w344 _] -> w270
      tunnel: [_ _ _ _ w353] -> w269
      tunnel: [_ _ _ _ w351] -> w268
      tunnel: w267 -> [_ w326 _ _ _]
      tunnel: w266 -> [_ _ w334 _ _]
      tunnel: w265 -> [_ _ _ w342 _]
      tunnel: w264 -> [_ _ _ _ w350]
      frame #0 {
        w319 = 16 ("y")
        n97 = Unbundle(w317) -> ("Array"=w316:dbl[])  [unwired: 4 out]
        n98 = Increment(x=w322) -> (x+1=w325:i32)
        n99 = Replace Array Subset(array=w316, new element=w323, index=w322) -> (w321:dbl[])
        n100 = Add Array Elements(numeric array=w321) -> (sum=w320:dbl)
        n101 = Quotient & Remainder(x=w325, y=w319) -> (x-y*floor(x/y)=w324:i32)  [unwired: 1 out]
        n102 = Divide(x=w320, y=w319) -> (x/y=w318:dbl)
      }
      frame #1 {
        n103 = Unbundle(w328) -> ("Array 2"=w327:dbl[])  [unwired: 4 out]
        n104 = Replace Array Subset(array=w327, new element=w326, index=w333) -> (w329:dbl[])
        n105 = Add Array Elements(numeric array=w329) -> (sum=w332:dbl)
        n106 = Divide(x=w332, y=16) -> (x/y=w330:dbl)
      }
      frame #2 {
        n107 = Unbundle(w338) -> ("Array 3"=w335:dbl[])  [unwired: 4 out]
        n108 = Replace Array Subset(array=w335, new element=w334, index=w341) -> (w336:dbl[])
        n109 = Add Array Elements(numeric array=w336) -> (sum=w340:dbl)
        n110 = Divide(x=w340, y=16) -> (x/y=w337:dbl)
      }
      frame #3 {
        n111 = Unbundle(w346) -> ("Array 4"=w343:dbl[])  [unwired: 4 out]
        n112 = Replace Array Subset(array=w343, new element=w342, index=w349) -> (w345:dbl[])
        n113 = Add Array Elements(numeric array=w345) -> (sum=w348:dbl)
        n114 = Divide(x=w348, y=16) -> (x/y=w344:dbl)
      }
      frame #4 {
        n115 = Unbundle(w354) -> ("Array 5"=w352:dbl[])  [unwired: 4 out]
        n116 = Replace Array Subset(array=w352, new element=w350, index=w357) -> (w353:dbl[])
        n117 = Add Array Elements(numeric array=w353) -> (sum=w356:dbl)
        n118 = Divide(x=w356, y=16) -> (x/y=w351:dbl)
      }
    }
    n119 = Bundle(w279, w277, w273, w270, w268) -> (w297:cluster{dbl, dbl, dbl, dbl, dbl})  [unwired: 1 in]
    "Flow Rate" <- w297
    n120 = Bundle("Array"=w278, "Array 2"=w276, "Array 3"=w272, "Array 4"=w271, "Array 5"=w269) -> (w275:T11)  [unwired: 1 in]
    n121 = call "DAQ Assistant2"() -> ("data"=w262:dynamicdata)  [unwired: 17 in, 2 out]
    n122 = case shown="False" w310 {
      tunnel: [_ w558] -> w312
      frame False {
      }
      frame True {
        n123 = call "Dresser DXD Temp and Press Read Standalone.vi"("Serial Port (COM1)"="Pressure COM", "DXD Address (1)"=T16 2, "Pressure Units (PSI)"="Unit") -> ("Current Pressure"=w552:dbl, "Current Temperature"=w555:dbl)  [unwired: 9 in, 2 out]
        n124 = call "Dresser DXD Temp and Press Read Standalone.vi"("Serial Port (COM1)"="Pressure COM", "DXD Address (1)"=T16 2, "Pressure Units (PSI)"="Unit") -> ("Current Pressure"=w553:dbl, "Current Temperature"=w551:dbl)  [unwired: 9 in, 2 out]
        n125 = call "Dresser DXD Temp and Press Read Standalone.vi"("Serial Port (COM1)"="Pressure COM", "DXD Address (1)"=T16 3, "Pressure Units (PSI)"="Unit") -> ("Current Pressure"=w554:dbl, "Current Temperature"=w550:dbl)  [unwired: 9 in, 2 out]
        n126 = call "Dresser DXD Temp and Press Read Standalone.vi"("Serial Port (COM1)"="Pressure COM", "DXD Address (1)"=T16 4, "Pressure Units (PSI)"="Unit") -> ("Current Pressure"=w556:dbl, "Current Temperature"=w549:dbl)  [unwired: 9 in, 2 out]
        n127 = Bundle("Current Pressure"=w552, "Current Pressure"=w553, "Current Pressure"=w554, "Current Pressure"=w556) -> (w558:T5)  [unwired: 1 in]
        "Pressure" <- w558
        n128 = Bundle("Current Temperature"=w555, "Current Temperature"=w551, "Current Temperature"=w550, "Current Temperature"=w549) -> (→"Temp":T4)  [unwired: 1 in]
      }
    }
    n129 = call "Convert from Dynamic Data2"("Dynamic Data Type"=w262) -> ("Array"=w303:dbl[])  [unwired: 3 in]
    n130 = Index Array(array=w303, index=0) -> (element=w306:dbl)
    n131 = Index Array(array=w303, index=1) -> (element=w305:dbl)
    n132 = Index Array(array=w303, index=2) -> (element=w304:dbl)
    n133 = Bundle(w306, w305, w304) -> (→"Thermocouple T-Plots":cluster{dbl, dbl, dbl})  [unwired: 1 in]
    n134 = local read "Data Cluster 2"() -> (w260:T1)
    "Data Cluster 2" <- w260
    n135 = case shown="True" "Collect Spectra" {
      tunnel: w294 -> [_ w382]
      tunnel: [_ w383] -> w293
      tunnel: w291 -> [_ w383]
      tunnel: [_ w359] -> w289
      tunnel: [_ w366] -> w288
      tunnel: w287 -> [_ w381]
      tunnel: [_ w377] -> w286
      tunnel: w285 -> [_ w380]
      frame False {
        # "Not importing Raman spectra from the RXN4 computer"
      }
      frame True {
        n136 = Subtract(x=w383, y=w382) -> (x-y=w386:i32)
        n137 = Equal?(x=w386, y=1) -> (x = y?=w384:bool)
        n138 = stacked-sequence {
          tunnel: w384 -> [w422 w449 w476 w503]
          tunnel: [w417 _ _ _] -> w370
          tunnel: w381 -> [w421 w448 w475 w502]
          tunnel: [w420 _ _ _] -> w378
          tunnel: w380 -> [w419 w447 w474 w501]
          tunnel: [w418 _ _ _] -> w371
          tunnel: [_ w446 _ _] -> w379
          tunnel: [_ w444 _ _] -> w369
          tunnel: [_ w445 _ _] -> w376
          tunnel: [_ _ w473 _] -> w375
          tunnel: [_ _ w471 _] -> w368
          tunnel: [_ _ w472 _] -> w374
          tunnel: [_ _ _ w500] -> w373
          tunnel: [_ _ _ w498] -> w367
          tunnel: [_ _ _ w499] -> w372
          tunnel: TRUE ("Default File Path or Specify? (T = specify)") -> [w416 w443 w470 w497]
          frame #0 {
            n139 = case shown="True" w422 {
              tunnel: [w426 w442] -> w418
              tunnel: [w424 w437] -> w417
              tunnel: [w425 w441] -> w420
              tunnel: w421 -> [_ w436]
              tunnel: w419 -> [_ w440]
              tunnel: w416 -> [w423 _]
              frame False {
                n140 = stacked-sequence {
                  seq-local: [w427 _] -> [_ w433]
                  tunnel: [w427 _] -> w424
                  tunnel: [_ w435] -> w426
                  tunnel: [_ w434] -> w425
                  tunnel: w423 -> [w428 _]
                  frame #0 {
                    n141 = case shown="True" w428 {
                      tunnel: [path "\\\\RXN3\\Users/11084/Desktop/FDA CFR Raman Data/TEST/RCT1/Grams" ("start path") w431] -> w427
                      frame False {
                      }
                      frame True {
                        n142 = call "File Dialog2"("start path"=path "C:/", "prompt"="Select Reactant 1 Data Folder") -> ("selected path"=w431:path)  [unwired: 10 in, 3 out]
                      }
                    }
                  }
                  frame #1 {
                    n143 = call "FileWatcher_SPCReader_FDA_v3.vi"("appended path"=w433) -> ("Filesnames out"=w434:string[], "Raman Spectrum"=w435:cluster{i32[], i32[]})  [unwired: 1 in]
                  }
                }
              }
              frame True {
                n144 = Unbundle(w436) -> ("selected path"=w437:path)  [unwired: 3 out]
                n145 = Index Array(array=w440, index (row)=0) -> (element=w438:string[])  [unwired: 1 in]
                n146 = call "FileWatcher_SPCReader_FDA_v3.vi"("Filenames in"=w438, "appended path"=w437) -> ("Filesnames out"=w441:string[], "Raman Spectrum"=w442:cluster{i32[], i32[]})
              }
            }
          }
          frame #1 {
            n147 = case shown="True" w449 {
              tunnel: [w453 w469] -> w446
              tunnel: [w451 w464] -> w444
              tunnel: [w452 w468] -> w445
              tunnel: w448 -> [_ w463]
              tunnel: w447 -> [_ w466]
              tunnel: w443 -> [w450 _]
              frame False {
                n148 = stacked-sequence {
                  seq-local: [w454 _] -> [_ w460]
                  tunnel: [w454 _] -> w451
                  tunnel: [_ w462] -> w453
                  tunnel: [_ w461] -> w452
                  tunnel: w450 -> [w455 _]
                  frame #0 {
                    n149 = case shown="False" w455 {
                      tunnel: [path "\\\\RXN3\\Users/11084/Desktop/FDA CFR Raman Data/TEST/RCT2/Grams" ("start path") w458] -> w454
                      frame False {
                      }
                      frame True {
                        n150 = call "File Dialog3"("start path"=path "C:/", "prompt"="Select Reactant 2 Data Folder") -> ("selected path"=w458:path)  [unwired: 10 in, 3 out]
                      }
                    }
                  }
                  frame #1 {
                    n151 = call "FileWatcher_SPCReader_FDA_v3.vi"("appended path"=w460) -> ("Filesnames out"=w461:string[], "Raman Spectrum"=w462:cluster{i32[], i32[]})  [unwired: 1 in]
                  }
                }
              }
              frame True {
                n152 = Unbundle(w463) -> ("selected path"=w464:path)  [unwired: 3 out]
                n153 = Index Array(array=w466, index (row)=1) -> (element=w465:string[])  [unwired: 1 in]
                n154 = call "FileWatcher_SPCReader_FDA_v3.vi"("Filenames in"=w465, "appended path"=w464) -> ("Filesnames out"=w468:string[], "Raman Spectrum"=w469:cluster{i32[], i32[]})
              }
            }
          }
          frame #2 {
            n155 = case shown="False" w476 {
              tunnel: [w480 w496] -> w473
              tunnel: [w478 w490] -> w471
              tunnel: [w479 w495] -> w472
              tunnel: w475 -> [_ w491]
              tunnel: w474 -> [_ w493]
              tunnel: w470 -> [w477 _]
              frame False {
                n156 = stacked-sequence {
                  seq-local: [w481 _] -> [_ w487]
                  tunnel: [w481 _] -> w478
                  tunnel: [_ w489] -> w480
                  tunnel: [_ w488] -> w479
                  tunnel: w477 -> [w482 _]
                  frame #0 {
                    n157 = case shown="False" w482 {
                      tunnel: [path "\\\\RXN3\\Users/11084/Desktop/FDA CFR Raman Data/TEST/RCT3/Grams" ("start path") w485] -> w481
                      frame False {
                      }
                      frame True {
                        n158 = call "File Dialog4"("start path"=path "C:/", "prompt"="Select Reactant 3 Data Folder") -> ("selected path"=w485:path)  [unwired: 10 in, 3 out]
                      }
                    }
                  }
                  frame #1 {
                    n159 = call "FileWatcher_SPCReader_FDA_v3.vi"("appended path"=w487) -> ("Filesnames out"=w488:string[], "Raman Spectrum"=w489:cluster{i32[], i32[]})  [unwired: 1 in]
                  }
                }
              }
              frame True {
                n160 = Unbundle(w491) -> ("selected path"=w490:path)  [unwired: 3 out]
                n161 = Index Array(array=w493, index (row)=2) -> (element=w492:string[])  [unwired: 1 in]
                n162 = call "FileWatcher_SPCReader_FDA_v3.vi"("Filenames in"=w492, "appended path"=w490) -> ("Filesnames out"=w495:string[], "Raman Spectrum"=w496:cluster{i32[], i32[]})
              }
            }
          }
          frame #3 {
            n163 = case shown="True" w503 {
              tunnel: [w507 w523] -> w500
              tunnel: [w505 w517] -> w498
              tunnel: [w506 w522] -> w499
              tunnel: w502 -> [_ w518]
              tunnel: w501 -> [_ w520]
              tunnel: w497 -> [w504 _]
              frame False {
                n164 = stacked-sequence {
                  seq-local: [w508 _] -> [_ w514]
                  tunnel: [w508 _] -> w505
                  tunnel: [_ w516] -> w507
                  tunnel: [_ w515] -> w506
                  tunnel: w504 -> [w509 _]
                  frame #0 {
                    n165 = case shown="False" w509 {
                      tunnel: [path "\\\\RXN3\\Users/11084/Desktop/FDA CFR Raman Data/TEST/PRD1/Grams" ("start path") w512] -> w508
                      frame False {
                      }
                      frame True {
                        n166 = call "File Dialog5"("start path"=path "C:/", "prompt"="SelectProduct Data Folder") -> ("selected path"=w512:path)  [unwired: 10 in, 3 out]
                      }
                    }
                  }
                  frame #1 {
                    n167 = call "FileWatcher_SPCReader_FDA_v3.vi"("appended path"=w514) -> ("Filesnames out"=w515:string[], "Raman Spectrum"=w516:cluster{i32[], i32[]})  [unwired: 1 in]
                  }
                }
              }
              frame True {
                n168 = Unbundle(w518) -> ("selected path"=w517:path)  [unwired: 3 out]
                n169 = Index Array(array=w520, index (row)=3) -> (element=w519:string[])  [unwired: 1 in]
                n170 = call "FileWatcher_SPCReader_FDA_v3.vi"("Filenames in"=w519, "appended path"=w517) -> ("Filesnames out"=w522:string[], "Raman Spectrum"=w523:cluster{i32[], i32[]})
              }
            }
          }
        }
        n171 = Build Array(w371, w379, w375, w373) -> (w359:cluster{i32[], i32[]}[])
        n172 = Build Array(w378, w376, w374, w372) -> (w377:string[][])
        n173 = stacked-sequence {
          tunnel: w359 -> [w391 w398 w405 w412]
          tunnel: [w387 _ _ _] -> w364
          tunnel: [_ w394 _ _] -> w363
          tunnel: [_ _ w401 _] -> w362
          tunnel: [_ _ _ w408] -> w361
          frame #0 {
            n174 = Index Array(array=w391, index=0) -> (element=w390:cluster{i32[], i32[]})
            n175 = Unbundle(w390) -> (w389:i32[])  [unwired: 1 out]
            n176 = Add Array Elements(numeric array=w389) -> (sum=w392:i32)
            n177 = Not Equal?(x=w392, y=0) -> (x != y?=w387:bool)
          }
          frame #1 {
            n178 = Index Array(array=w398, index=1) -> (element=w397:cluster{i32[], i32[]})
            n179 = Unbundle(w397) -> (w396:i32[])  [unwired: 1 out]
            n180 = Add Array Elements(numeric array=w396) -> (sum=w399:i32)
            n181 = Not Equal?(x=w399, y=0) -> (x != y?=w394:bool)
          }
          frame #2 {
            n182 = Index Array(array=w405, index=2) -> (element=w404:cluster{i32[], i32[]})
            n183 = Unbundle(w404) -> (w403:i32[])  [unwired: 1 out]
            n184 = Add Array Elements(numeric array=w403) -> (sum=w406:i32)
            n185 = Not Equal?(x=w406, y=0) -> (x != y?=w401:bool)
          }
          frame #3 {
            n186 = Index Array(array=w412, index=3) -> (element=w411:cluster{i32[], i32[]})
            n187 = Unbundle(w411) -> (w410:i32[])  [unwired: 1 out]
            n188 = Add Array Elements(numeric array=w410) -> (sum=w413:i32)
            n189 = Not Equal?(x=w413, y=0) -> (x != y?=w408:bool)
          }
        }
        n190 = Bundle("selected path"=w370, "selected path"=w369, "selected path"=w368, "selected path"=w367) -> (w366:T9)  [unwired: 1 in]
        "Raman Data Path" <- w366
        n191 = Build Array(w364, w363, w362, w361) -> (w360:bool[])
        n192 = Or Array Elements(Boolean array=w360) -> (logical OR=w365:bool)
        n193 = case shown="True" w365 {
          tunnel: w359 -> [_ w415]
          frame False {
          }
          frame True {
            "Raman Spectrum" <- w415
          }
        }
      }
    }
    n194 = case shown="True" "Write to File?" {
      tunnel: w262 -> [_ w548]
      tunnel: w312 -> [_ w547]
      tunnel: w297 -> [_ w546]
      tunnel: w291 -> [_ w541]
      tunnel: w290 -> [_ w540]
      tunnel: [w524 w538] -> w296
      tunnel: w281 -> [w524 w542]
      tunnel: [_ w541] -> w292
      tunnel: w289 -> [_ w539]
      tunnel: w284 -> [_ w532]
      tunnel: w261 -> [_ w531]
      tunnel: w260 -> [_ w525]
      frame False {
        # "eventually find more elegant way\nto do this - currently just an output on/off\nswitch for all intents and purposes"
      }
      frame True {
        n195 = Subtract(x=w541, y=w540) -> (x-y=w545:i32)
        n196 = Equal?(x=w545, y=1) -> (x = y?=w543:bool)
        n197 = call "File_Write_v2.vi"("Thermocouple Data"=w548, "Pressure Data"=w547, 2:w525, "Flow Rate Data"=w546, "Raman Data Array"=w539, "Loop Iteration Boolean"=w543, "File Path Cluster"=w542, "Numeric"=w531, "Array"=w532) -> (14:"Data_noRaman path"=w533:path, 15:"Data_Reactant 1 path"=→"Data_Reactant 1 path":path, 16:"Data_Reactant 1 path"=w534:path, 17:"Data_Reactant 2 path"=→"Data_Reactant 2 path":path, 20:"Data_Reactant 2 path"=w535:path, 21:"Data_Reactant 3 path"=w536:path, 23:"Data_Product path"=→"Data_Product path":path, 24:"Data_noRaman path"=→"Data_noRaman path":path, 25:"Data_Product path"=w537:path, 27:"Data_Reactant 3 path"=→"Data_Reactant 3 path":path)  [unwired: 9 in]
        n198 = Bundle("Data_noRaman path"=w533, "Data_Reactant 1 path"=w534, "Data_Reactant 2 path"=w535, "Data_Reactant 3 path"=w536, "Data_Product path"=w537) -> (w538:T17)  [unwired: 1 in]
      }
    }
  }
  n199 = Release Queue(queue=w14) -> ()  [unwired: 2 in, 3 out]
  n200 = property on="Temp" class="WFChart (strict)"("History Data"=T15 []) -> ()  [unwired: 2 in, 2 out]
  n201 = property on="Pressure" class="WFChart (strict)"("History Data"=T14 []) -> ()  [unwired: 2 in, 2 out]
  n202 = property on="Thermocouple T-Plots" class="WFChart (strict)"("History Data"=cluster{dbl, dbl, dbl}[] []) -> ()  [unwired: 2 in, 2 out]
  n203 = property on="Flow Rate" class="WFChart (strict)"("History Data"=T12 []) -> ()  [unwired: 2 in, 2 out]
  n204 = property on="Raman Spectrum" class="XYGraph (strict)"("Value"=cluster{i32[], i32[]}[] [] ("Raman Spectrum")) -> ()  [unwired: 2 in, 2 out]
